vi "Export Configuration RTM.vi"(8 "error in (no error)":errorcluster, 11 "Node Ptr":u64 format="%.0x") -> (0 "error out":errorcluster)   [LabVIEW 2017, in "Routing and Faulting System Explorer.lvlib"]
uses:
  Routing and Faulting System Explorer.lvlib
  Shared/Import Export/Import Export.lvlib
panel:
  in  "Tag":string
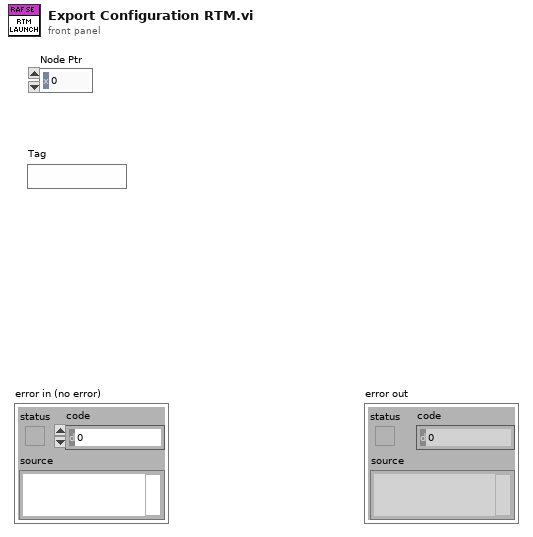
[diagram p1: front panel]
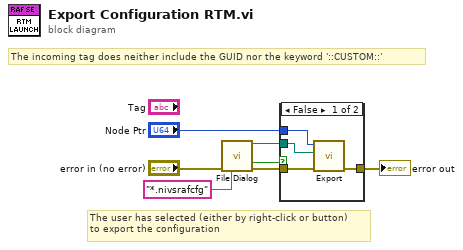
[diagram p0: block diagram]
diagram:
  # "The user has selected (either by right-click or button)\nto export the configuration"
  # "The incoming tag does neither include the GUID nor the keyword '::CUSTOM::'"
  n1 = call "File Dialog"("error in"="error in (no error)", "pattern (all files)"="*.nivsrafcfg") -> ("selected path"=w1:path, "cancelled"=w5:bool, "error out"=w4:errorcluster)  [unwired: 10 in, 1 out]
  n2 = case shown="False" w5 {
    tunnel: w4 -> [w11 w12]
    tunnel: [w10 w12] -> w3
    tunnel: "Node Ptr" -> [w9 _]
    tunnel: w1 -> [w8 _]
    frame False {
      n3 = call "Export.vi"("error in"=w11, "path"=w8, "item in"=w9) -> ("error out"=w10:errorcluster)  [unwired: 7 in, 1 out]
    }
    frame True {
    }
  }
  "error out" <- w3
